vi "Init Analysis Graphs 1.vi"(4 "Shots":u32=125, 6 "Image Size":cluster{"Height":u32, "Width":u32}={"Height"=480, "Width"=640}, 7 "Z - Time Signal":refnum<vi>, 9 "Signal Map Analysis":refnum<vi>, 10 "Intensity Width Graph Analysis":refnum<vi>, 11 "Intensity Height Graph Analysis":refnum<vi>) -> (0 "error out":errorcluster, 3 "Analysis Graph out":refnum<class "Graph with Analysis Controls.lvclass">)   [LabVIEW 2023, in "test Init Analysis Graph.lvclass"]
uses:
  test Init Analysis Graph.lvclass
  test Init Analysis Graph.lvclass/test Init Analysis Graph.ctl
  source/Analysis Graph/Graph with Analysis Controls.lvclass
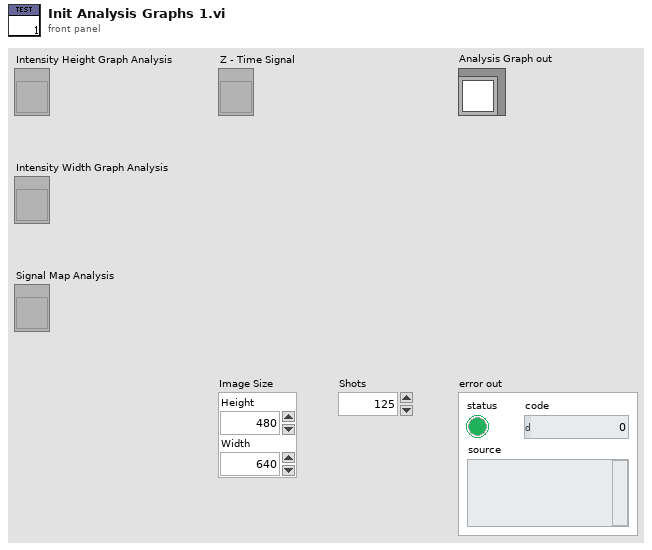
[diagram p1: front panel]
types:
  T1 = cluster{"Z-Graph Ref":refnum<vi>, "Graph Ref":refnum<vi>, "Y-Graph Ref":refnum<vi>, "X-Graph Ref":refnum<vi>}
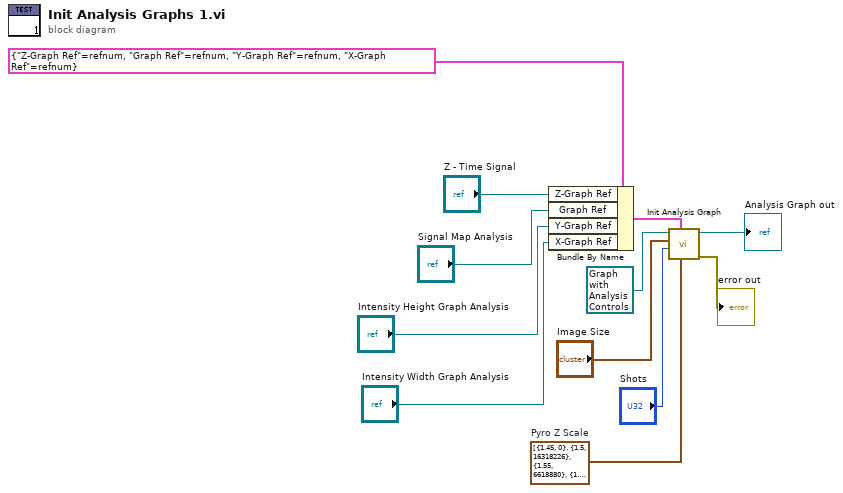
[diagram p0: block diagram]
diagram:
  w1 = cluster{"Numeric":dbl, "Color Box":u32}[] [{"Numeric"=1.45, "Color Box"=0}, {"Numeric"=1.5, "Color Box"=16318226}, {"Numeric"=1.55, "Color Box"=6618880}, {"Numeric"=1.6, "Color Box"=1507583}, {"Numeric"=1.65, "Color Box"=16711680}, {"Numeric"=1.7, "Color Box"=16448250}]  # Pyro Z Scale
  n1 = Bundle By Name(cluster=T1 {"Z-Graph Ref"=refnum, "Graph Ref"=refnum, "Y-Graph Ref"=refnum, "X-Graph Ref"=refnum} ("Graphs"), "Z-Graph Ref"="Z - Time Signal", "Graph Ref"="Signal Map Analysis", "Y-Graph Ref"="Intensity Height Graph Analysis", "X-Graph Ref"="Intensity Width Graph Analysis") -> (w5:T1)
  n2 = call "Init Analysis Graph.vi"("Z Scale.Marker Values[]"=w1, "Graphs"=w5, "Shots"="Shots", "Image Size"="Image Size", "Analysis Graph in"=refnum<class "Graph with Analysis Controls.lvclass"> refnum) -> ("error out"=→"error out":errorcluster, "Analysis Graph out"=→"Analysis Graph out":refnum<class "Graph with Analysis Controls.lvclass">)  [unwired: 5 in]
